vi "Cluster to gRPC LabVIEW Message.vi"(7 "Package Name":string, 8 "error in":errorcluster, 11 "Cluster":variant) -> (0 "error out":errorcluster, 2 "gRPC Enum Metadata out":T1[](array[typedef]), 3 "gRPC Message Metadata []":T2[](array[typedef]))   [LabVIEW 2019, in "grpc-lvsupport.lvlib"]
uses:
  grpc-lvsupport.lvlib
  typeDefs/Message Metadata.ctl
  typeDefs/Message Element Metadata.ctl
  typeDefs/Message Element Type.ctl
  typeDefs/Enum Metadata.ctl
  <vilib>/Utility/Data Type/NI_Data Type.lvlib
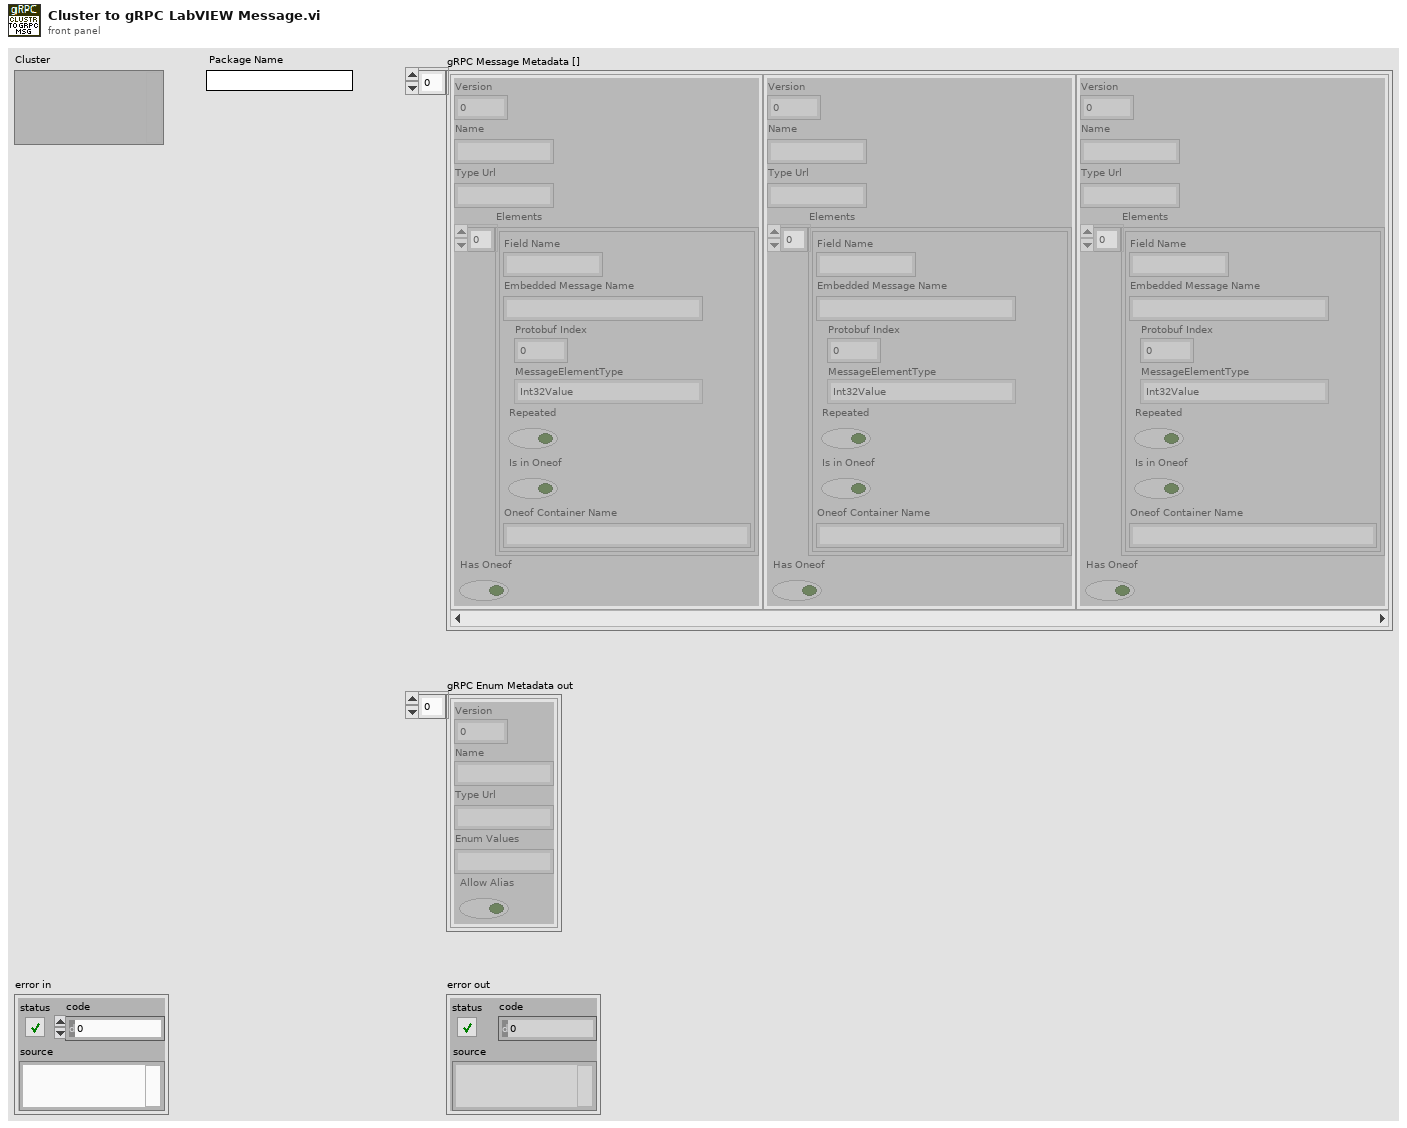
[diagram p1: front panel]
types:
  T1 = typedef "grpc-lvsupport.lvlib/Enum Metadata.ctl" = cluster{"Version":i32, "Name":string, "Type Url":string, "Enum Values":string, "Allow Alias":bool}
  T2 = typedef "grpc-lvsupport.lvlib/Message Metadata.ctl" = cluster{"Version":i32, "Name":string, "Type Url":string, "Elements":T3[], "Has Oneof":bool}
  T3 = typedef "grpc-lvsupport.lvlib/Message Element Metadata.ctl" = cluster{"Field Name":string, "Embedded Message Name":string, "Protobuf Index":i32, "MessageElementType":T4, "Repeated":bool, "Is in Oneof":bool, "Oneof Container Name":string}
  T4 = typedef "grpc-lvsupport.lvlib/Message Element Type.ctl" = enum32{"Int32Value", "FloatValue", "DoubleValue", "BoolValue", "StringValue", "MessageValue", "Int64Value", "UInt32Value", "UInt64Value", "EnumValue", "Bytes", "Fixed64", "Fixed32", "SFixed64", "SFixed32", "SInt64", "SInt32"}
  T5 = typedef "NI_Data Type.lvlib/Data Type.ctl" = enum8{"Invalid Type", "Void", "I8", "I16", "I32", "I64", "U8", "U16", "U32", "U64", "Single Float", "Double Float", "Extended Float", "Single Complex", "Double Complex", "Extended Complex", "Enum U8", "Enum U16", "Enum U32", "Enum U64", "Single Float With Unit", "Double Float With Unit", "Extended Float With Unit", "Single Complex with Unit", "Double Complex with Unit", "Extended Complex with Unit", "Boolean", "String", "Path", "Picture", "Tag", "Array", "Cluster", "Variant", "LV Variant", "Waveform", "Timestamp", "Digital Waveform", "Digital Data", "ExpressData", "Refnum", "External Data", "VI", "Poly VI", "LabVIEW Class Instance", "Fixed Point", "Set Collection", "Map Collection"}
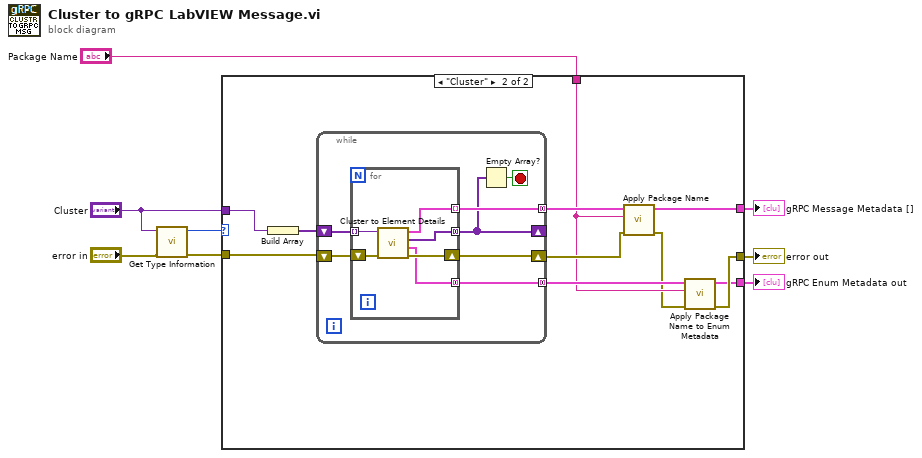
[diagram p0: block diagram]
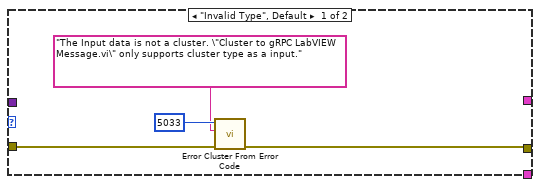
[diagram p2: hidden frame]
diagram:
  n1 = call <vilib>:"Get Type Information.vi"("error in (no error)"="error in", "variant"="Cluster") -> ("error out"=w6:errorcluster, "type"=w3:T5)  [unwired: 5 in, 3 out]
  n2 = case shown="\"Cluster\"" w3 {
    tunnel: [_ w19] -> w5
    tunnel: [w11 w14] -> w8
    tunnel: "Package Name" -> [_ w16]
    tunnel: w6 -> [w12 w22]
    tunnel: "Cluster" -> [_ w18]
    tunnel: [_ w13] -> w1
    frame "Invalid Type", Default {
      n3 = call <vilib>:"Error Cluster From Error Code.vi"("error in (no error)"=w12, "error message (\"\")"="The Input data is not a cluster. \"Cluster to gRPC LabVIEW Message.vi\" only supports cluster type as a input." ("error message (\"\")"), "error code (0)"=5033) -> ("error out"=w11:errorcluster)  [unwired: 6 in]
    }
    frame "Cluster" {
      n4 = Build Array(w18) -> (w21:variant[])
      n5 = while {
        shift-right: [w25] -> _
        shift-left: w21 -> [w28]
        tunnel: [w27] -> w20 mode=concatenating
        shift-right: [w30] -> w23
        shift-left: w22 -> [w29]
        tunnel: [w24] -> w17 mode=concatenating
        stop <- w26 stop-if-true
        n6 = for {
          tunnel: [w34] -> w25 mode=concatenating
          tunnel: w28 -> [w33] mode=indexing
          tunnel: [w32] -> w27 mode=indexing
          shift-right: [w36] -> w30
          shift-left: w29 -> [w35]
          tunnel: [w31] -> w24 mode=concatenating
          n7 = call "Cluster to Element Details.vi"("error in"=w35, "Cluster"=w33) -> ("error out"=w36:errorcluster, "gRPC Enum Metadata"=w31:T1[], "More Cluster"=w34:variant[], "gRPC Message Metadata"=w32:T2)  [unwired: 6 in]
        }
        n8 = Empty Array?(array=w25) -> (empty?=w26:bool)
      }
      n9 = call "Apply Package Name.vi"("error in"=w23, "Package Name"=w16, "gRPC Message Metadata in"=w20) -> ("error out"=w15:errorcluster, "gRPC Message Metadata"=w19:T2[])  [unwired: 7 in]
      n10 = call "Apply Package Name to Enum Metadata.vi"("error in"=w15, "Package Name"=w16, "gRPC Enum Metadata in"=w17) -> ("error out"=w14:errorcluster, "gRPC Enum Metadata out"=w13:T1[])  [unwired: 7 in]
    }
  }
  "gRPC Message Metadata []" <- w5
  "error out" <- w8
  "gRPC Enum Metadata out" <- w1
